vi "freqToVolt.vi"(1 "频率":dbl) -> (0 "电压":dbl)   [LabVIEW 2018]
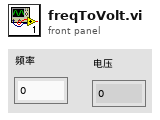
[diagram p1: front panel]
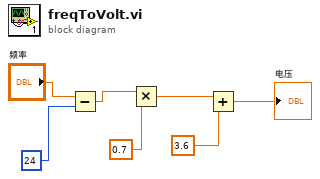
[diagram p0: block diagram]
diagram:
  n1 = Subtract(x="频率", y=24) -> (x-y=w4:dbl)
  n2 = Multiply(x=w4, y=0.7) -> (x*y=w3:dbl)
  n3 = Add(x=w3, y=3.6) -> (x+y=→"电压":dbl)
